vi "Time Frequency Average.vi"(0 "Y":dbl[](array[numeric]), 5 "Time avgs":i32, 7 "Freq avgs":i32=1, 9 "Npts":i32, 11 "error in (no error)":errorcluster, 12 "df (kHz)":dbl) -> (4 "Ave waveform":dbl[](array[numeric]), 6 "Averaged Spectrum (Vrms)":dbl[](array[numeric]), 8 "waveform cluster":cluster{i32, "dx":dbl, "Array":dbl[]}, 10 "Complex Spectrum":cdb[](array[numeric]), 15 "error out":errorcluster)   [LabVIEW 2020]
uses:
  977e999b-1b92-443b-be85-17ed600b82f4.vi
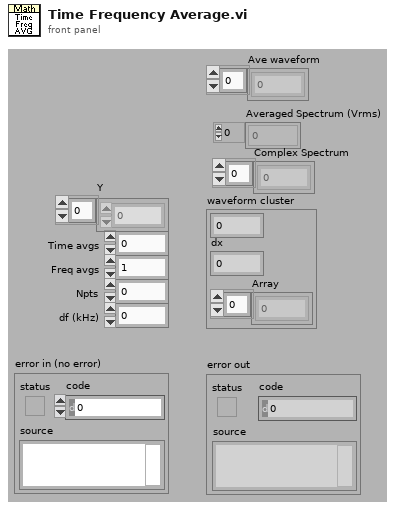
[diagram p1: front panel]
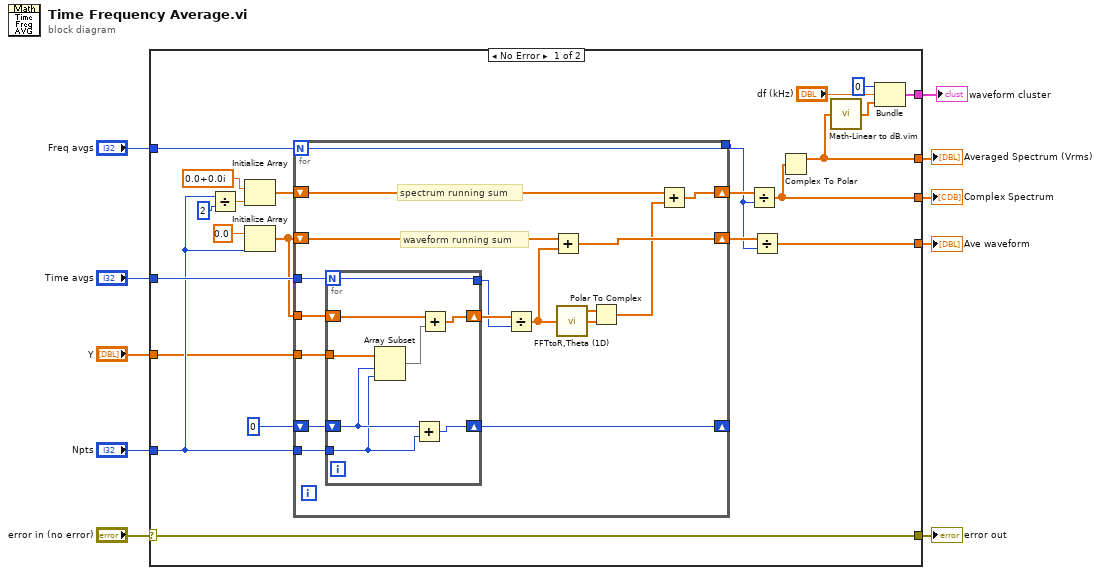
[diagram p0: block diagram]
diagram:
  n1 = case shown="No Error" "error in (no error)" {
    selector: "error in (no error)" -> [w16 w58]
    tunnel: "Freq avgs" -> [w13 _]
    tunnel: "Time avgs" -> [w29 _]
    tunnel: "Y" -> [w15 _]
    tunnel: "Npts" -> [w25 _]
    tunnel: [w12 _] -> w6
    tunnel: [w14 _] -> w5
    tunnel: [w17 _] -> w4
    tunnel: [w16 w58] -> w2
    tunnel: [w11 _] -> w1
    frame No Error {
      n2 = Divide(x=w25, y=2) -> (x/y=w30:dbl)
      n3 = Initialize Array(cdb 0.0+0.0i, w30) -> (w26:cdb[])
      n4 = Initialize Array(0.0, w25) -> (w27:dbl[])
      n5 = for {
        N: w13 -> [w36]
        shift-right: [w48] -> w23
        shift-left: w26 -> [w49]
        shift-right: [w46] -> w22
        shift-left: w27 -> [w47]
        tunnel: w27 -> [w45]
        tunnel: w29 -> [w42]
        tunnel: w15 -> [w41]
        tunnel: w25 -> [w40]
        shift-right: [w37] -> _
        shift-left: 0 -> [w39]
        tunnel: [w36] -> w21
        # "spectrum running sum"
        # "waveform running sum"
        n6 = for {
          N: w42 -> [w51]
          shift-right: [w56] -> w44
          shift-left: w45 -> [w57]
          tunnel: w41 -> [w55]
          tunnel: w40 -> [w53]
          shift-right: [w52] -> w37
          shift-left: w39 -> [w54]
          tunnel: [w51] -> w38
          n7 = Array Subset(array=w55, index=w54, length=w53) -> (w50:dbl[])
          n8 = Add(x=w54, y=w53) -> (x+y=w52:i32)
          n9 = Add(x=w57, y=w50) -> (x+y=w56:dbl[])
        }
        n10 = Divide(x=w44, y=w38) -> (x/y=w43:dbl[])
        n11 = Add(x=w47, y=w43) -> (x+y=w46:dbl[])
        n12 = call "FFTtoR,Theta (1D).VI"("X"=w43) -> ("+Freq. Mag of FFT"=w35:dbl[], "+Freq Theta of FFT"=w34:dbl[])  [unwired: 1 in]
        n13 = Polar To Complex(1:w34, 2:w35) -> (0:w33:cdb[])
        n14 = Add(x=w49, y=w33) -> (x+y=w48:cdb[])
      }
      n15 = Divide(x=w23, y=w21) -> (x/y=w11:cdb[])
      n16 = Divide(x=w22, y=w21) -> (x/y=w14:dbl[])
      n17 = Complex To Polar(r * e^(i*theta)=w11) -> (r=w12:dbl[])  [unwired: 1 out]
      n18 = call "Math-Linear to dB.vim"("linear"=w12) -> ("dB"=w18:dbl[])
      n19 = Bundle(0, "df (kHz)"="df (kHz)", "dB"=w18) -> (w17:cluster{i32, "df (kHz)":dbl, "dB":dbl[]})  [unwired: 1 in]
    }
    frame Error {
    }
  }
  "error out" <- w2
  "Averaged Spectrum (Vrms)" <- w6
  "waveform cluster" <- w4
  "Ave waveform" <- w5
  "Complex Spectrum" <- w1
